vi "TDMS path settings updated.vi"(8 "error in":errorcluster, 10 "Settings":T1={"TDMS Filepath"=path "", "TDMS Directory"=path "", "Dir?"=TRUE}) -> (0 "error out":errorcluster)   [LabVIEW 2019, in "Filepath Editor.lvlib"]
doc: "Updated file path settings for reading\n_____\nCreated using DQMH Event Scripter 6.1.0.128."
uses:
  Filepath Editor.lvlib
  Settings--cluster.ctl
  TDMS path settings updated Argument--cluster.ctl
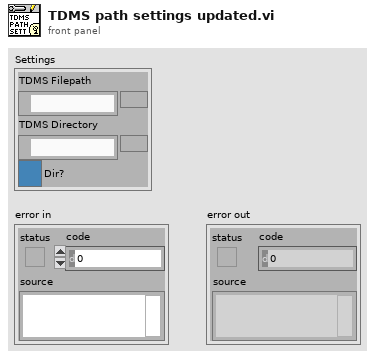
[diagram p1: front panel]
types:
  T1 = typedef "Filepath Editor.lvlib/Settings--cluster.ctl" = cluster{"TDMS Filepath":path, "TDMS Directory":path, "Dir?":bool}
  T2 = typedef "Filepath Editor.lvlib/TDMS path settings updated Argument--cluster.ctl" = cluster{"Settings":T1}
  T3 = typedef "Filepath Editor.lvlib/Broadcast Events--cluster.ctl" = cluster{"Module Did Init":refnum<user-event>, "Status Updated":refnum<user-event>, "Error Reported":refnum<user-event>, "Module Did Stop":refnum<user-event>, "Update Module Execution Status":refnum<user-event>, "TDMS path settings updated":refnum<user-event>}
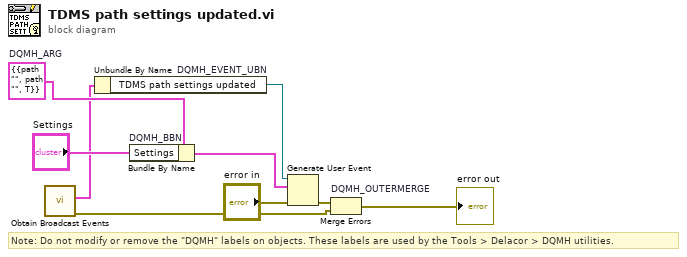
[diagram p0: block diagram]
diagram:
  w4 = T2 {"Settings"={"TDMS Filepath"=path "", "TDMS Directory"=path "", "Dir?"=TRUE}}  # DQMH_ARG
  # "Note: Do not modify or remove the \"DQMH\" labels on objects. These labels are used by the Tools > Delacor > DQMH utilities."
  n1 = call "Obtain Broadcast Events.vi"() -> ("error out"=w2:errorcluster, "Filepath Editor Broadcast Events"=w1:T3)  [unwired: 10 in]
  n2 = Unbundle By Name "DQMH_EVENT_UBN"(w1) -> ("TDMS path settings updated"=w6:refnum<user-event>)
  n3 = Bundle By Name "DQMH_BBN"(cluster=w4, "Settings"="Settings") -> (w7:T2)
  n4 = Generate User Event(user event=w6, event data cluster=w7, error in="error in") -> (error out=w5:errorcluster)  [unwired: 1 in, 1 out]
  n5 = Merge Errors "DQMH_OUTERMERGE"(w5, w2) -> (→"error out":errorcluster)
